vi "GetVIRefnum.vi"(8 "error in (no error)":errorcluster, 11 "object in":refnum<class "Vi_Button.lvclass">) -> (0 "error out":errorcluster, 2 "VI Refnum":refnum<vi>, 3 "object out":refnum<class "Vi_Button.lvclass">)   [LabVIEW 2018, in "Vi_Button.lvclass"]
uses:
  Vi_Button.lvclass
panel:
  # "https://www.google.co.uk/search?q=alternatives+to+remmina&ie=utf-8&oe=utf-8&meta=cr%3DcountryUK|countryGB#hl=en&cr=countryUK|countryGB&tbs=ctr:countryUK|countryGB&sclient=psy-ab&q=vinagre+rdp&oq=vinagre+rdp&gs_l=serp.3..0l3j0i30.6251.6812.1.7098.4.4.0.0.0.0.77.298.4.4.0.les%3B..0.0...1c.1.4.psy-ab.YOcOaR-SSD4&pbx=1&bav=on.2,or.r_gc.r_pw.r_cp.r_qf.&bvm=bv.42768644,d.d2k&fp=d936680fd2fddaac&biw=1680&bih=808"
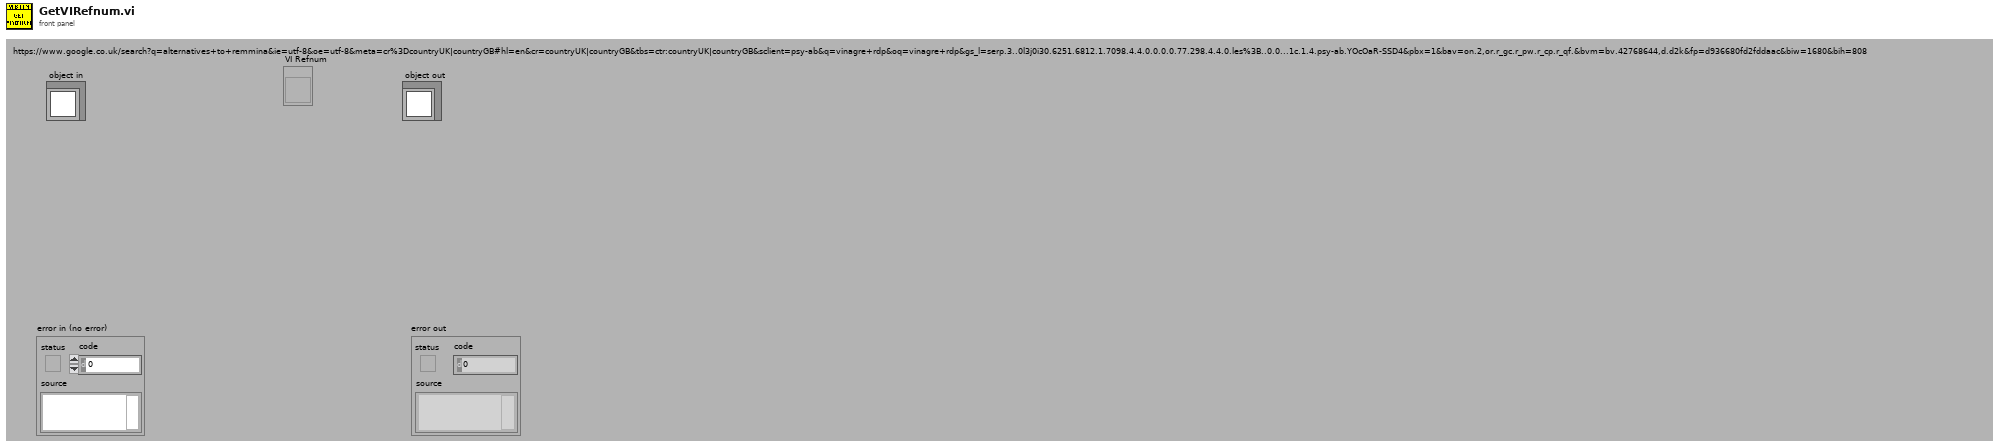
[diagram p1: front panel]
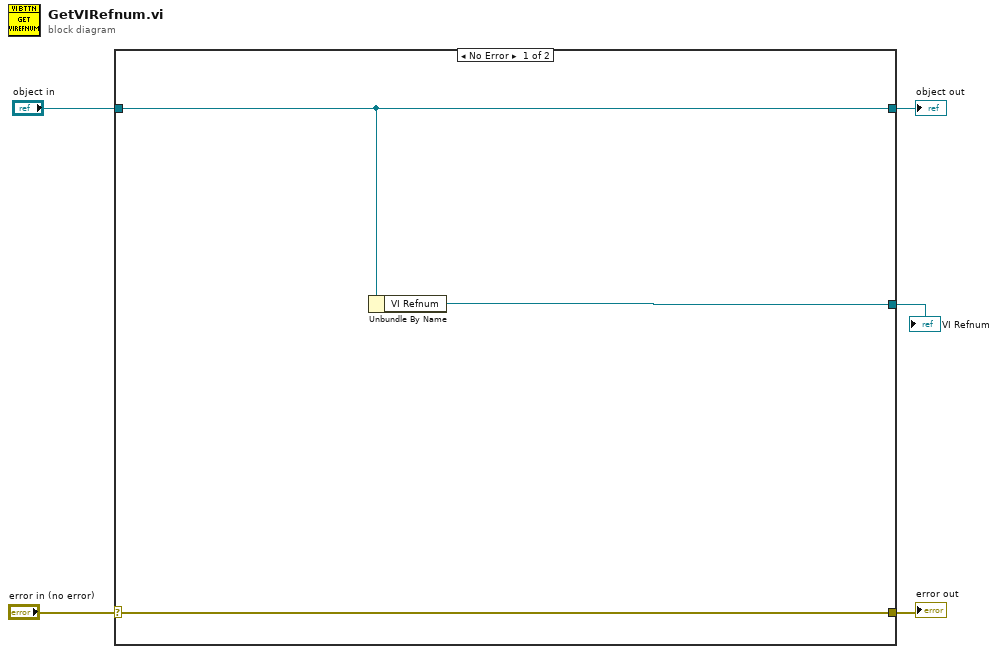
[diagram p0: block diagram]
diagram:
  n1 = case shown="No Error" "error in (no error)" {
    selector: "error in (no error)" -> [w7 w10]
    tunnel: [w7 w10] -> w4
    tunnel: [w6 w9] -> w2
    tunnel: "object in" -> [w6 w9]
    tunnel: [w8 _] -> w1
    frame No Error {
      n2 = Unbundle By Name(w6) -> ("VI Refnum"=w8:refnum<vi>)
    }
    frame Error {
    }
  }
  "error out" <- w4
  "object out" <- w2
  "VI Refnum" <- w1
